vi "PH_ImageOperator.publish Statistician Data.vi"(0 "i ref in":refnum<vi>, 5 "error in":errorcluster) -> (14 "i ref out":refnum<vi>, 19 "error out":errorcluster)   [LabVIEW 2014, in "PH_ImageOperator.lvlib"]
doc: "This VI is forseen to publish the statistician data via DIM."
uses:
  PH_ImageOperator.lvlib
  PH_ImageStatistician/PH_ImageStatistician.Statistician Data.ctl
  CSlibraries-extern/DimLVEvent/LVDimInterface/LVDimInterface.lvlib
  PH_ImageStatistician/PH_ImageStatistician.lvlib
panel:
  in  "Statistician Data":T1
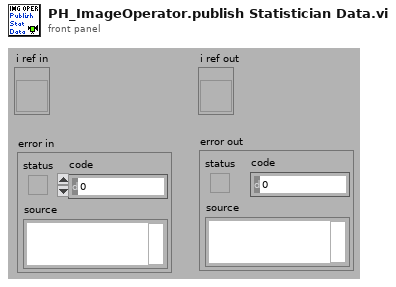
[diagram p1: front panel]
types:
  T1 = typedef "PH_ImageStatistician.lvlib/PH_ImageStatistician.Statistician Data.ctl" = cluster{"Snapshot Time":dbl, "Maj FWHM":dbl, "Min FWHM":dbl, "Maj Fit Order":dbl, "Min Fit Order":dbl, "99% Diam Maj Trace":dbl, "99% Diam Min Trace":dbl, "Theta":dbl, "Delta":dbl, "Maj Diam":dbl, "Min Diam":dbl, "Azimuth Angle":dbl, "Azi Angle rel to major?":dbl, "Ellipticity":dbl, "CoG - X":dbl, "CoG - Y":dbl, "Energy":dbl, "Energy Cal - no mJ":dbl, "Lin Cal - no mm or mrad":dbl, "Lin Cal Factor":dbl}
  T2 = typedef "PH_ImageOperator.lvlib/PH_ImageOperator.i attribute.ctl" = cluster{"GUI Refs":cluster{"Delete":refnum<vi>, "Calibration status":refnum<vi>, "BI subtracted":refnum<vi>, "calc Energy":refnum<vi>, "Energy: expected value":refnum<vi>, "Energy: Tolerance":refnum<vi>, "Energy calculated":refnum<vi>, "Energy":refnum<vi>, "calc Beam Anal":refnum<vi>, "Maj Diam 1/esquare":refnum<vi>, "Min Diam 1/esquare":refnum<vi>, "Azi Angle":refnum<vi>, "Min/Maj Diam esquare":refnum<vi>, "Beam analysed":refnum<vi>, "CoG - x":refnum<vi>, "CoG - y":refnum<vi>, "BA: Method":refnum<vi>, "BA: Steps":refnum<vi>, "BA: Factor":refnum<vi>, "calc Traces":refnum<vi>, "Traces: Fit Gauss":refnum<vi>, "Traces calculated":refnum<vi>, "Maj FWHM":refnum<vi>, "Min FWHM":refnum<vi>, "Major Trace":refnum<vi>, "Minor Trace":refnum<vi>, "Maj Fit Order":refnum<vi>, "Min Fit Order":refnum<vi>, "Position calculated":refnum<vi>, "Position":refnum<vi>, "Type":refnum<vi>, "Center":refnum<vi>, "exp - X":refnum<vi>, "exp - Y":refnum<vi>, "Tolerance":refnum<vi>, "f":refnum<vi>, "M":refnum<vi>, "D":refnum<vi>, "q":refnum<vi>, "Dummy Method":refnum<vi>, "Dummy Type":refnum<vi>, "Global On":refnum<vi>, "Traces: No offset":refnum<vi>, "Maj 99%":refnum<vi>, "Min 99%":refnum<vi>, "GUI FF Image":refnum<vi>, "calc Fill Factor":refnum<vi>, "FF calculated":refnum<vi>, "Fill Factor: Filter?":refnum<vi>, "FF: Damage Threshold":refnum<vi>, "FF: Threshold":refnum<vi>, "FF: max allow. Energy":refnum<vi>, "FF: Fillfactor":refnum<vi>, "Calibration data":refnum<vi>}, "List of GUIs":string[], "Calibration":cluster{"Status":T3, "Calibration data":T4, "Calibration Data File":path}, "Final Image":cluster{"BI Subtraction Failure":bool}, "Energy":cluster{"on":bool, "expected value [mJ]":dbl, "Tolerance [%]":dbl, "State":T3, "Energy [mJ]":dbl, "Unit":string, "calculated @":timestamp}, "Beam Analysis":cluster{"on":bool, "Data":T5, "Method":bool, "Steps":i32, "Factor":i32, "ROI":cluster{"Left":i32, "Top":i32, "Right":i32, "Bottom":i32}, "analysed @":timestamp}, "Trace Analysis":cluster{"on":bool, "Fit on":bool, "Maj FWHM":dbl, "Min FWHM":dbl, "Maj Fit Order":i32, "Min Fit Order":i32, "No Offset":bool, "Maj 99%":dbl, "Min 99%":dbl, "Traces":cluster{"XScaleName":string, "Y Scale Minimum":sgl, "Y Scale Maximum":sgl, "X Scale Minimum":sgl, "X Scale Maximum":sgl, "Traces":cluster{"Index":sgl[], "Trace":dbl[]}[]}[], "analysed @":timestamp}, "Position Analysis":cluster{"on":bool, "exp - X":i32, "exp - Y":i32, "focal length [mm]":dbl, "Magnification":dbl, "Delta":dbl, "Theta":dbl, "Tolerance":dbl, "Type":bool, "analysed @":timestamp}, "Fill Factor":cluster{"on":bool, "Filter on?":bool, "Threshold":dbl, "Damage Threshold [J/cm²]":dbl, "Fillfactor":dbl, "Max. allowed Energy [J]":dbl, "calculated @":timestamp}, "Statistician Service ID":i32, "Images":cluster{"Background":T6, "OP":T6, "GUI":T6, "BA: ROI":T6, "Trace: Turn":T6, "FF: Main":T6, "FF: Help":T6, "PSDB: BG":T6, "PSDB: OP":T6, "PSDB: FF":T6}}
  T3 = typedef "PH_StatusHandler.lvlib/PH_StatusHandler.Status.ctl" = i16
  T4 = typedef "PH_ImageCalibrator.lvlib/PH_ImageCalibrator.Calibration Data.ctl" = cluster{"Date":string, "Time":string, "Cam Settings":cluster{"Cam ID":string, "Gain":dbl, "Brightness":dbl, "Shutter":dbl, "Cam Error":bool, "Mode":i32}, "Background Image":cluster{"Image":dbl[][], "Image Error":bool}, "Linear Calibration":cluster{"Calibration Factor":dbl, "not mm or mrad":bool}, "Energy Calibration":cluster{"Calibration Factor":dbl, "no mJ":bool}}
  T5 = typedef "PH_ImageOperator.lvlib/PH_ImageOperator.Beam Analysis Data.ctl" = cluster{"CoG-x":sgl, "CoG-y":sgl, "Maj Dim":dbl, "Min Dim":dbl, "Ellipticity":dbl, "Azimuth Angle [rad]":dbl, "Azi Angle rel to Maj?":bool}
  T6 = typedef "IMAQ Image.ctl" = refnum<image>
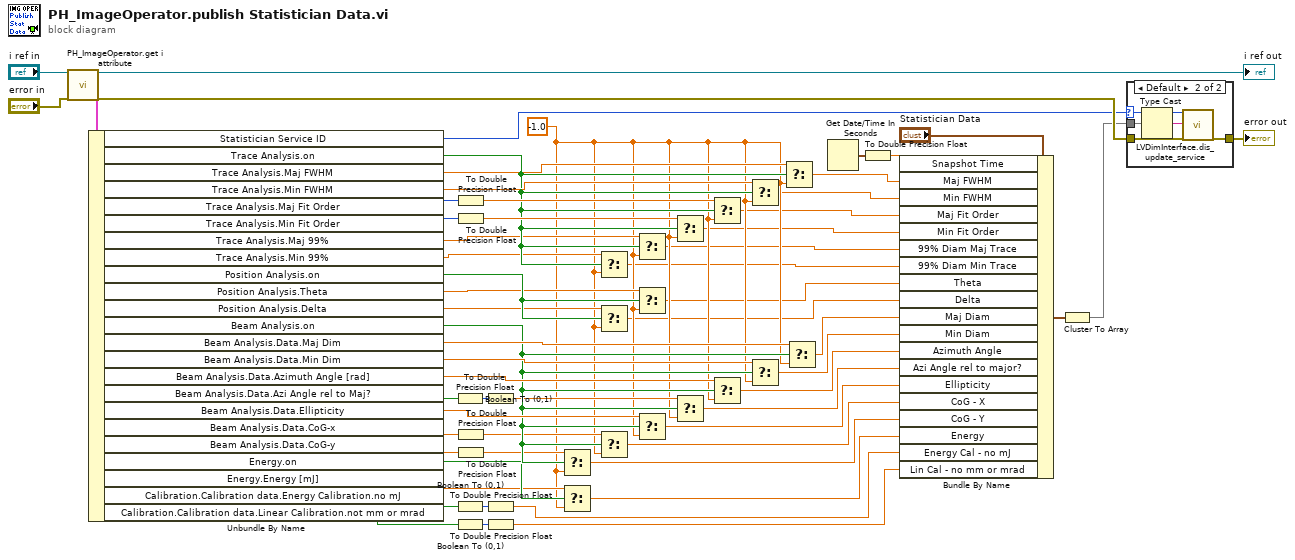
[diagram p0: block diagram]
diagram:
  w31 = -1.0 ("element")
  n1 = call "PH_ImageOperator.get i attribute.vi"("i ref in"="i ref in", "error in (no error)"="error in") -> ("i ref out"=→"i ref out":refnum<vi>, "i attribute"=w58:T2, "error out"=w30:errorcluster)  [unwired: 15 in]
  n2 = Unbundle By Name(w58) -> ("Statistician Service ID"=w28:i32, "Trace Analysis.on"=w51:bool, "Trace Analysis.Maj FWHM"=w57:dbl, "Trace Analysis.Min FWHM"=w56:dbl, "Trace Analysis.Maj Fit Order"=w55:i32, "Trace Analysis.Min Fit Order"=w54:i32, "Trace Analysis.Maj 99%"=w50:dbl, "Trace Analysis.Min 99%"=w49:dbl, "Position Analysis.on"=w48:bool, "Position Analysis.Theta"=w47:dbl, "Position Analysis.Delta"=w46:dbl, "Beam Analysis.on"=w39:bool, "Beam Analysis.Data.Maj Dim"=w45:dbl, "Beam Analysis.Data.Min Dim"=w44:dbl, "Beam Analysis.Data.Azimuth Angle [rad]"=w43:dbl, "Beam Analysis.Data.Azi Angle rel to Maj?"=w36:bool, "Beam Analysis.Data.Ellipticity"=w42:dbl, "Beam Analysis.Data.CoG-x"=w41:sgl, "Beam Analysis.Data.CoG-y"=w40:sgl, "Energy.on"=w33:bool, "Energy.Energy [mJ]"=w32:dbl, "Calibration.Calibration data.Energy Calibration.no mJ"=w5:bool, "Calibration.Calibration data.Linear Calibration.not mm or mrad"=w3:bool)
  n3 = Boolean To (0,1)(Boolean=w36) -> (0, 1=w35:i16)
  n4 = Boolean To (0,1)(Boolean=w5) -> (0, 1=w6:i16)
  n5 = Boolean To (0,1)(Boolean=w3) -> (0, 1=w4:i16)
  n6 = To Double Precision Float(number=w55) -> (double precision float=w53:dbl)
  n7 = To Double Precision Float(number=w54) -> (double precision float=w52:dbl)
  n8 = To Double Precision Float(number=w41) -> (double precision float=w38:dbl)
  n9 = To Double Precision Float(number=w40) -> (double precision float=w37:dbl)
  n10 = To Double Precision Float(number=w35) -> (double precision float=w34:dbl)
  n11 = To Double Precision Float(number=w6) -> (double precision float=w2:dbl)
  n12 = To Double Precision Float(number=w4) -> (double precision float=w1:dbl)
  n13 = Select(t=w37, s=w39, f=w31) -> (s? t:f=w8:dbl)
  n14 = Select(t=w32, s=w33, f=w31) -> (s? t:f=w7:dbl)
  n15 = Select(t=w49, s=w51, f=w31) -> (s? t:f=w17:dbl)
  n16 = Select(t=w46, s=w48, f=w31) -> (s? t:f=w15:dbl)
  n17 = Select(t=w38, s=w39, f=w31) -> (s? t:f=w9:dbl)
  n18 = Select(t=w50, s=w51, f=w31) -> (s? t:f=w18:dbl)
  n19 = Select(t=w47, s=w48, f=w31) -> (s? t:f=w16:dbl)
  n20 = Select(t=w42, s=w39, f=w31) -> (s? t:f=w10:dbl)
  n21 = Select(t=w52, s=w51, f=w31) -> (s? t:f=w19:dbl)
  n22 = Select(t=w34, s=w39, f=w31) -> (s? t:f=w11:dbl)
  n23 = Select(t=w53, s=w51, f=w31) -> (s? t:f=w20:dbl)
  n24 = Select(t=w43, s=w39, f=w31) -> (s? t:f=w12:dbl)
  n25 = Select(t=w56, s=w51, f=w31) -> (s? t:f=w21:dbl)
  n26 = Select(t=w44, s=w39, f=w31) -> (s? t:f=w13:dbl)
  n27 = Select(t=w57, s=w51, f=w31) -> (s? t:f=w22:dbl)
  n28 = Select(t=w45, s=w39, f=w31) -> (s? t:f=w14:dbl)
  n29 = Get Date/Time In Seconds() -> (seconds since 1Jan1904=w26:timestamp)
  n30 = To Double Precision Float(number=w26) -> (double precision float=w25:dbl)
  n31 = Bundle By Name(cluster="Statistician Data", "Snapshot Time"=w25, "Maj FWHM"=w22, "Min FWHM"=w21, "Maj Fit Order"=w20, "Min Fit Order"=w19, "99% Diam Maj Trace"=w18, "99% Diam Min Trace"=w17, "Theta"=w16, "Delta"=w15, "Maj Diam"=w14, "Min Diam"=w13, "Azimuth Angle"=w12, "Azi Angle rel to major?"=w11, "Ellipticity"=w10, "CoG - X"=w9, "CoG - Y"=w8, "Energy"=w7, "Energy Cal - no mJ"=w2, "Lin Cal - no mm or mrad"=w1) -> (w24:T1)
  n32 = Cluster To Array(cluster=w24) -> (array=w23:dbl[])
  n33 = case shown="Default" w28 {
    selector: w28 -> [_ w63]
    tunnel: w23 -> [_ w66]
    tunnel: w30 -> [w62 w65]
    tunnel: [w62 w64] -> w29
    frame -1 {
    }
    frame Default {
      n34 = Type Cast(x=w66) -> (*(type *) &x=w67:string)  [unwired: 1 in]
      n35 = call "LVDimInterface.dis_update_service.vi"("my_serviceID"=w63, "data"=w67, "error in (no error)"=w65) -> ("error out"=w64:errorcluster)  [unwired: 14 in, 2 out]
    }
  }
  "error out" <- w29
